vi "Speaker Time Elapsed.vi"(8 "error in":errorcluster, 11 "cPAS in":refnum<class "cPAS.lvclass">) -> (0 "error out":errorcluster, 2 "TimeElapsed?":bool, 3 "cPAS out":refnum<class "cPAS.lvclass">)   [LabVIEW 2015, in "cPAS.lvclass"]
doc: "Check to see if the speaker time has elapsed. If it has, then send a signal to change the speaker position using the shared variables associated with the combined PAS-CRDS setup. This will occur in the next cycle."
uses:
  cPAS.lvclass
  Controls/Flags.ctl
  Reusable/PAS/Main/PAS.lvclass
  Reusable/Instrument/Instrument.lvclass
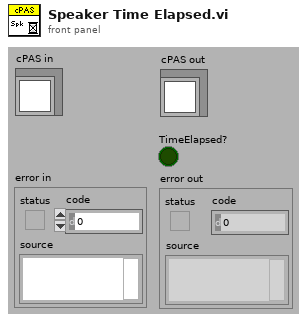
[diagram p1: front panel]
types:
  T1 = typedef "Flags.ctl" = enum8{"Autospeaker", "Link cycles", "Autofilter", "O3 Cal", "Filter Position"}
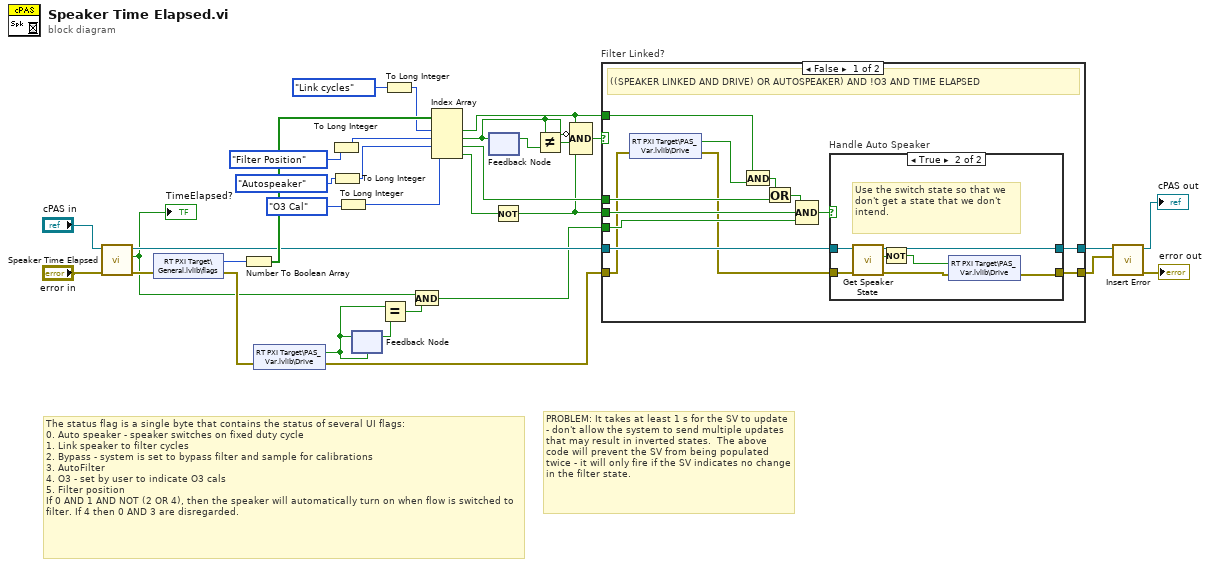
[diagram p0: block diagram]
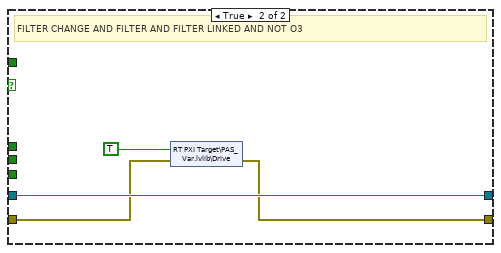
[diagram p3: hidden frame]
diagram:
  # "PROBLEM: It takes at least 1 s for the SV to update - don't allow the system to send multiple updates that may result in inverted states.  The above code will prevent the SV from being populated twice - it will only fire if the SV indicates no change in the filter state."
  # "The status flag is a single byte that contains the status of several UI flags: \n0. Auto speaker - speaker switches on fixed duty cycle \n1. Link speaker to filter cycles \n2. Bypass - system is set to bypass filter and sample for calibrations \n3. AutoFilter \n4. O3 - set by user to indicate O3 cals \n5. Filter position \nIf 0 AND 1 AND NOT (2 OR 4), then the speaker will automatically turn on when flow is switched to filter. If 4 then 0 AND 3 are disregarded."
  n1 = call-parent "Speaker Time Elapsed.vi"("error in"="error in", "PAS in"="cPAS in") -> ("error out"=w32:errorcluster, "TimeElapsed?"=w11:bool, "PAS out"=w24:refnum<class "cPAS.lvclass">)  [unwired: 7 in]
  "TimeElapsed?" <- w11
  n2 = shared-variable "RT PXI Target\\General.lvlib\\flags"(error in=w32) -> (w12:u8, error out=w17:errorcluster)
  n3 = Number To Boolean Array(number=w12) -> (Boolean array=w30:bool[])
  n4 = shared-variable "RT PXI Target\\PAS_Var.lvlib\\Drive"(error in=w17) -> (w13:bool, error out=w16:errorcluster)
  n5 = To Long Integer(number=Flags."Filter Position" ("Flags")) -> (32bit integer=w5:i32)
  n6 = To Long Integer(number=Flags."Autospeaker" ("Flags")) -> (32bit integer=w3:i32)
  n7 = To Long Integer(number=Flags."O3 Cal" ("Flags")) -> (32bit integer=w1:i32)
  n8 = feedback #1(w13) -> (w15:bool)
  n9 = feedback-in #1(w13) -> ()
  n10 = Equal?(x=w13, y=w15) -> (x = y?=w23:bool)
  n11 = To Long Integer(number=Flags."Link cycles" ("Flags")) -> (32bit integer=w7:i32)
  n12 = And(x=w11, y=w23) -> (x .and. y?=w22:bool)
  n13 = Index Array(array=w30, index #1=w7, index #2=w5, index #3=w3, index #4=w1) -> (element #1=w26:bool, element #2=w28:bool, element #3=w25:bool, element #4=w9:bool)
  n14 = feedback-in #2(w28) -> ()
  n15 = feedback #2() -> (w29:bool)  [unwired: 1 in]
  n16 = Not(x=w9) -> (.not. x?=w10:bool)
  n17 = Not Equal?(x=w28, y=w29) -> (x != y?=w31:bool)
  n18 = Compound Arithmetic op=AND(w26, invert w28, w31, w10) -> (w27:bool)
  n19 = case "Filter Linked?" shown="False" w27 {
    tunnel: [w46 w56] -> w21
    tunnel: w16 -> [w35 w57]
    tunnel: w26 -> [w42 _]
    tunnel: w22 -> [w39 _]
    tunnel: w10 -> [w40 _]
    tunnel: w25 -> [w41 _]
    tunnel: w24 -> [w38 w59]
    tunnel: [w37 w59] -> w20
    frame False {
      # "((SPEAKER LINKED AND DRIVE) OR AUTOSPEAKER) AND !O3 AND TIME ELAPSED"
      n20 = shared-variable "RT PXI Target\\PAS_Var.lvlib\\Drive"(error in=w35) -> (w36:bool, error out=w34:errorcluster)
      n21 = And(x=w42, y=w36) -> (x .and. y?=w45:bool)
      n22 = Or(x=w45, y=w41) -> (x .or. y?=w44:bool)
      n23 = Compound Arithmetic op=AND(w44, w40, w39) -> (w43:bool)
      n24 = case "Handle Auto Speaker" shown="True" w43 {
        tunnel: w34 -> [w48 w55]
        tunnel: [w48 w49] -> w46
        tunnel: w38 -> [w47 w54]
        tunnel: [w47 w52] -> w37
        frame False {
          # "On O3 or bypass"
        }
        frame True {
          # "Use the switch state so that we don't get a state that we don't intend."
          n25 = call "Get Speaker State.vi"("error in"=w55, "PAS in"=w54) -> ("error out"=w50:errorcluster, "State"=w53:bool, "PAS out"=w52:refnum<class "cPAS.lvclass">)  [unwired: 7 in]
          n26 = Not(x=w53) -> (.not. x?=w51:bool)
          n27 = shared-variable "RT PXI Target\\PAS_Var.lvlib\\Drive"(w51, error in=w50) -> (error out=w49:errorcluster)
        }
      }
    }
    frame True {
      # "FILTER CHANGE AND FILTER AND FILTER LINKED AND NOT O3"
      n28 = shared-variable "RT PXI Target\\PAS_Var.lvlib\\Drive"(TRUE ("drive"), error in=w57) -> (error out=w56:errorcluster)
    }
  }
  n29 = call "Insert Error.vi"("err"=w21, "Instrument in"=w20) -> ("error out"=→"error out":errorcluster, "Instrument out"=→"cPAS out":refnum<class "cPAS.lvclass">)  [unwired: 7 in, 1 out]
